vi "nes thing.vi"(1 "Y- Axis":dbl, 2 "X- Axis":dbl) -> (0 "Powah":dbl)   [LabVIEW 2012]
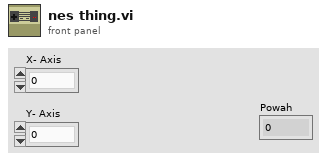
[diagram p1: front panel]
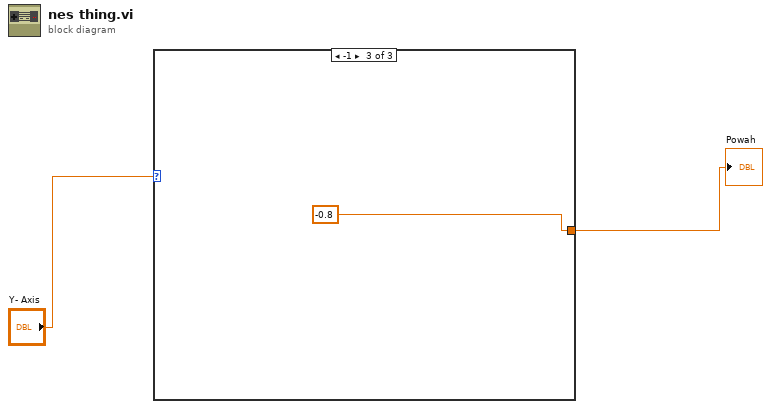
[diagram p0: block diagram]
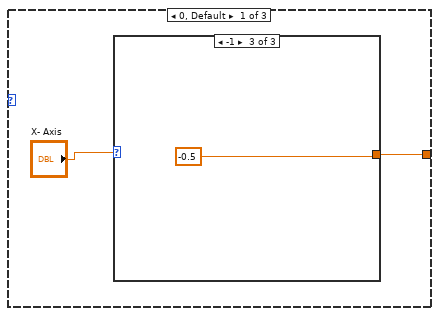
[diagram p2: hidden frame]
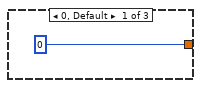
[diagram p3: hidden frame]
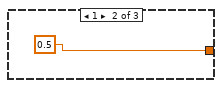
[diagram p4: hidden frame]
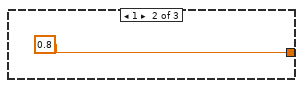
[diagram p5: hidden frame]
diagram:
  n1 = case shown="-1" "Y- Axis" {
    tunnel: [w3 0.8 -0.8] -> w1
    frame 0, Default {
      n2 = case shown="-1" "X- Axis" {
        tunnel: [0 0.5 -0.5] -> w3
        frame 0, Default {
        }
        frame 1 {
        }
        frame -1 {
        }
      }
    }
    frame 1 {
    }
    frame -1 {
    }
  }
  "Powah" <- w1
